vi "Transition.vi"(8 "error in (no error)":errorcluster, 9 "Milliseconds To Wait (-1, forever)":i32=-1, 10 "Target State Actor in":refnum<class "State Actor.lvclass">, 11 "State Actor in":refnum<class "State Actor.lvclass">) -> (0 "error out":errorcluster, 3 "State Actor out":refnum<class "State Actor.lvclass">)   [LabVIEW 2024, in "State Actor.lvlib" / "State Actor.lvclass"]
uses:
  State Actor.lvclass
  State Actor.lvclass/State Actor.ctl
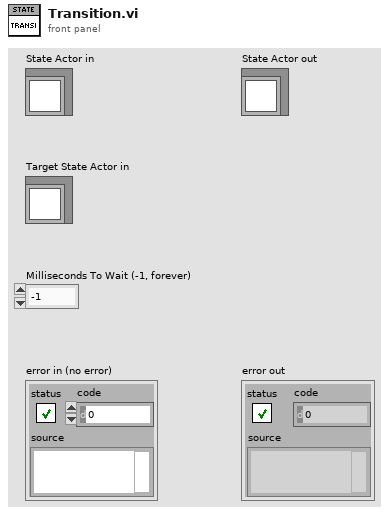
[diagram p1: front panel]
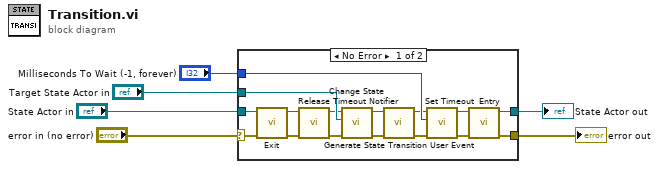
[diagram p0: block diagram]
diagram:
  n1 = case shown="No Error" "error in (no error)" {
    selector: "error in (no error)" -> [w22 w24]
    tunnel: [w18 w24] -> w5
    tunnel: [w19 w23] -> w3
    tunnel: "State Actor in" -> [w21 w23]
    tunnel: "Target State Actor in" -> [w20 _]
    tunnel: "Milliseconds To Wait (-1, forever)" -> [w15 _]
    frame No Error {
      n2 = call-dynamic "Exit.vi"("error in (no error)"=w22, "State Actor in"=w21) -> ("error out"=w12:errorcluster, "State Actor out"=w14:refnum<class "State Actor.lvclass">)  [unwired: 8 in]
      n3 = call "Release Timeout Notifier.vi"("error in (no error)"=w12, "State Actor in"=w14) -> ("error out"=w11:errorcluster, "State Actor out"=w13:refnum<class "State Actor.lvclass">)  [unwired: 8 in]
      n4 = call-dynamic "Change State.vi"("error in (no error)"=w11, "Target State Actor in"=w20, "State Actor in"=w13) -> ("error out"=w9:errorcluster, "State Actor out"=w10:refnum<class "State Actor.lvclass">)  [unwired: 7 in]
      n5 = call "Generate State Transition User Event.vi"("error in (no error)"=w9, "State Actor in"=w10) -> ("error out"=w8:errorcluster, "State Actor out"=w7:refnum<class "State Actor.lvclass">)  [unwired: 8 in]
      n6 = call "Set Timeout.vi"("error in (no error)"=w8, "Milliseconds To Wait (-1, forever)"=w15, "State Actor in"=w7) -> ("error out"=w16:errorcluster, "State Actor out"=w17:refnum<class "State Actor.lvclass">)  [unwired: 7 in]
      n7 = call-dynamic "Entry.vi"("error in (no error)"=w16, "State Actor in"=w17) -> ("error out"=w18:errorcluster, "State Actor out"=w19:refnum<class "State Actor.lvclass">)  [unwired: 8 in]
    }
    frame Error {
    }
  }
  "error out" <- w5
  "State Actor out" <- w3
